vi "GetCountFrom1ListCtrl.vi"(11 "ArrayRef in":refnum<vi>) -> (2 "result":i32, 3 "ArrayRef out":refnum<vi>)   [LabVIEW 2018, in "Library-Ctrl.lvlib"]
uses:
  Library-Ctrl.lvlib
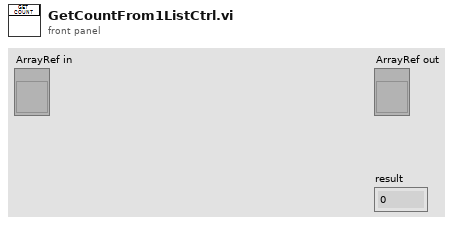
[diagram p1: front panel]
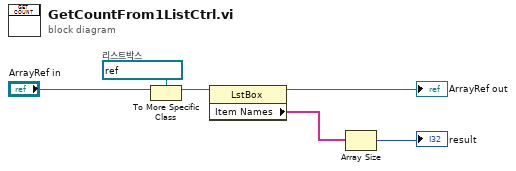
[diagram p0: block diagram]
diagram:
  w5 = refnum<vi> refnum  # 리스트박스
  n1 = To More Specific Class(target class=w5, reference="ArrayRef in") -> (specific class reference=w3:refnum<vi>)  [unwired: 1 in, 1 out]
  n2 = property class="LstBox"(reference=w3) -> (reference out=→"ArrayRef out":refnum<vi>, "Item Names"=w2:string[])  [unwired: 1 in, 1 out]
  n3 = Array Size(array=w2) -> (size(s)=→"result":i32)
